vi "simpletrigger.vi"() -> ()   [LabVIEW 2012]
uses:
  <vilib>/_DAQmxBase/Internals/DAQmxBase Create Channel (AI-Voltage-Basic).vi
  <vilib>/_DAQmxBase/Internals/DAQmxBase Timing (Sample Clock).vi
  <vilib>/_DAQmxBase/Internals/DAQmxBase Read (Analog 2D DBL NChan NSamp).vi
  <vilib>/_DAQmxBase/Internals/DAQmxBase Start Trigger (Analog Edge).vi
panel:
  in  "Trigger":bool
  out "Waveform Graph":dbl[][](graph) caption="Measurement"
  in  "level":dbl format="%0.2f"
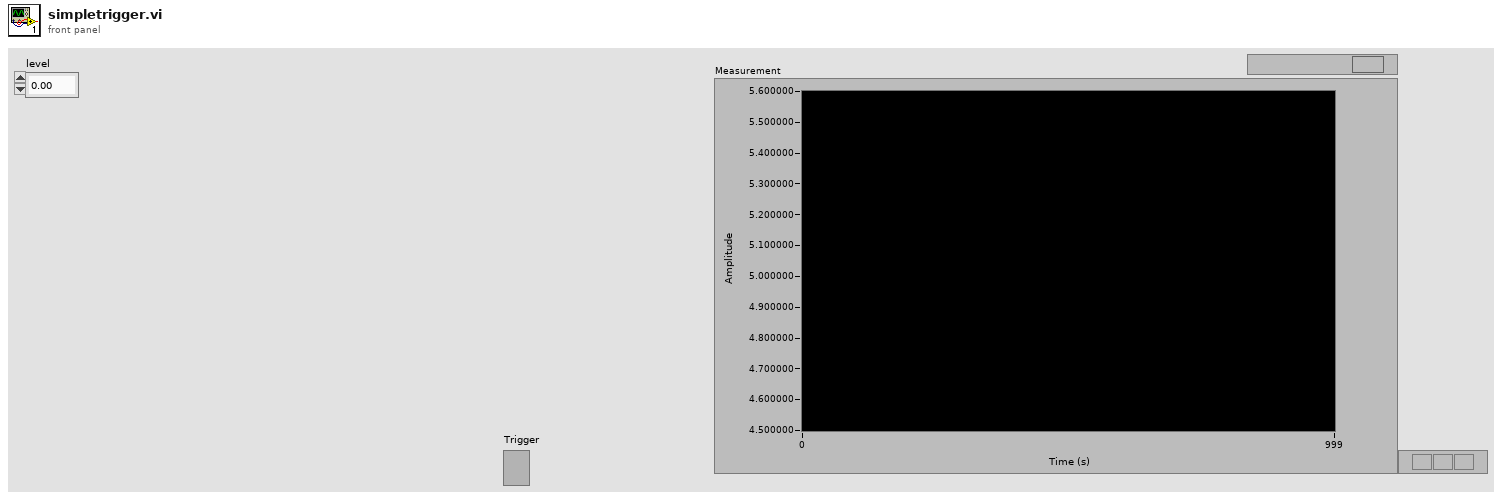
[diagram p1: front panel]
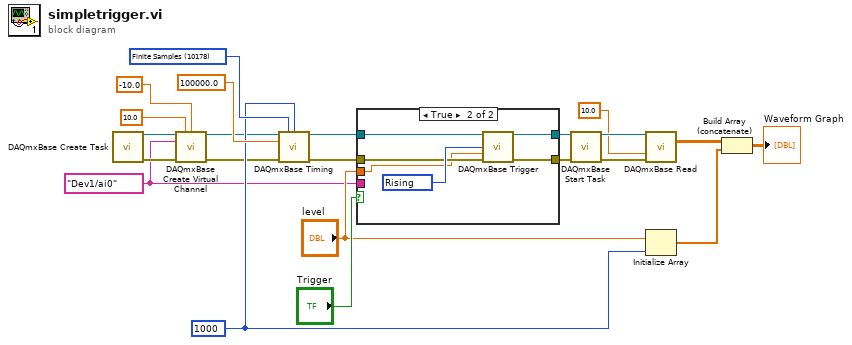
[diagram p0: block diagram]
diagram:
  w1 = tag "Dev1/ai0" ("DAQmx Physical Channel")
  w4 = 1000 ("samples per channel")
  w22 = 10178 items=["Finite Samples"=10178, "Continuous Samples"=10123] ("sample mode")
  n1 = call <vilib>:"DAQmxBase Create Task.vi"() -> ("task out"=w18:refnum<k21>, "error out"=w17:errorcluster)  [unwired: 14 in]
  n2 = call-poly <vilib>:"DAQmxBase Create Virtual Channel.vi"("task in"=w18, "maximum value"=10.0, "minimum value"=-10.0, "physical channels"=w1, "error in"=w17) -> ("task out"=w3:refnum<k21>, "error out"=w2:errorcluster)  [unwired: 9 in]
  n3 = call-poly <vilib>:"DAQmxBase Timing.vi"("task/channels in"=w3, "sample mode"=w22, "samples per channel"=w4, "rate"=100000.0, "error in"=w2) -> ("task out"=w16:refnum<k21>, "error out"=w15:errorcluster)  [unwired: 2 in, 7 out]
  n4 = case shown="True" "Trigger" {
    tunnel: w16 -> [w24 w25]
    tunnel: w15 -> [w23 w29]
    tunnel: [w24 w28] -> w14
    tunnel: [w23 w27] -> w13
    tunnel: "level" -> [_ w26]
    tunnel: w1 -> [_ _]
    frame False {
    }
    frame True {
      w30 = 10280 items=["Rising"=10280, "Falling"=10171] ("slope")
      n5 = call-poly <vilib>:"DAQmxBase Trigger.vi"("task/channels in"=w25, "slope"=w30, "level"=w26, "error in"=w29) -> ("task out"=w28:refnum<k21>, "error out"=w27:errorcluster)  [unwired: 10 in]
    }
  }
  n6 = call <vilib>:"DAQmxBase Start Task.vi"("task/channels in"=w14, "error in"=w13) -> ("task out"=w21:refnum<k21>, "error out"=w20:errorcluster)  [unwired: 12 out]
  n7 = call-poly <vilib>:"DAQmxBase Read.vi"("task/channels in"=w21, "timeout"=10.0, "error in"=w20) -> ("data"=w6:dbl[][])  [unwired: 10 in, 2 out]
  n8 = Initialize Array("level", w4) -> (w7:dbl[])
  n9 = Build Array (concatenate)(w6, w7) -> (→"Waveform Graph":dbl[][])
